vi "Image To Clipboard.vi"(8 "error in (no error)":errorcluster, 11 "24-bit pixmap":u32[][](array[numeric]) format="%x") -> (0 "error out":errorcluster)   [LabVIEW 2023, in "LV-Awesome.lvlib"]
uses:
  System.Drawing
  System.Windows.Forms
  LV-Awesome.lvlib
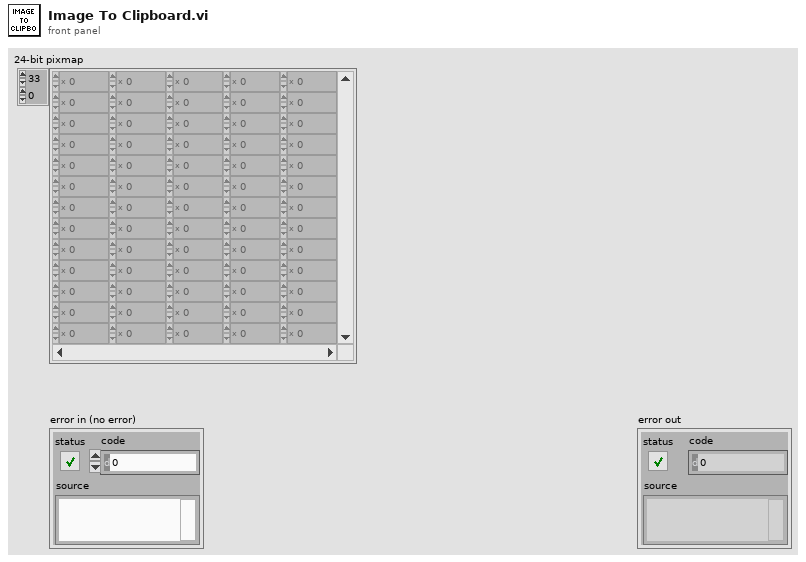
[diagram p1: front panel]
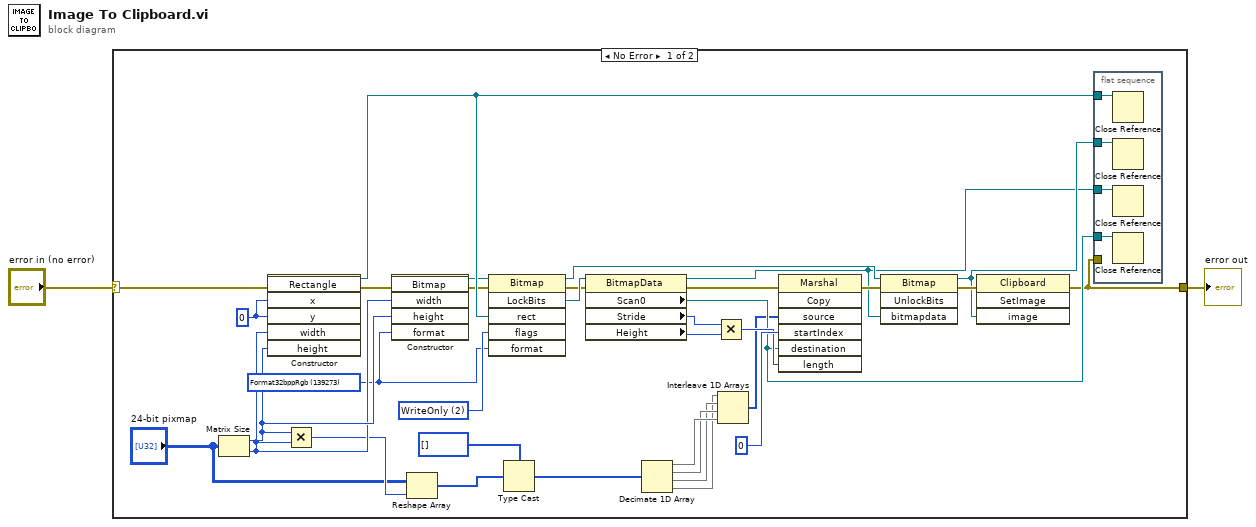
[diagram p0: block diagram]
diagram:
  n1 = case shown="No Error" "error in (no error)" {
    selector: "error in (no error)" -> [w11 w41]
    tunnel: [w10 w41] -> w1
    frame No Error {
      w35 = 2 items=["ReadOnly"=1, "WriteOnly"=2, "ReadWrite"=3, "UserInputBuffer"=4] ("flags")
      w36 = 0 ("x")
      w20 = 139273 items=["DontCare, Undefined"=0, "Max"=15, "Indexed"=65536, "Gdi"=131072, "Format16bppRgb555"=135173, "Format16bppRgb565"=135174, "Format24bppRgb"=137224, "Format32bppRgb"=139273, "Format1bppIndexed"=196865, "Format4bppIndexed"=197634, "Format8bppIndexed"=198659, "Alpha"=262144, "Format16bppArgb1555"=397319, "PAlpha"=524288, "Format32bppPArgb"=925707, "Extended"=1048576, "Format16bppGrayScale"=1052676, "Format48bppRgb"=1060876, "Format64bppPArgb"=1851406, "Canonical"=2097152, "Format32bppArgb"=2498570, "Format64bppArgb"=3424269] ("format")
      n2 = Matrix Size(0:"24-bit pixmap") -> (1:w32:i32, 2:w31:i32)
      n3 = constructor class="Rectangle"(error in=w11, "x"=w36, "y"=w36, "width"=w31, "height"=w32) -> (reference out=w13:refnum<k24>, error out=w25:errorcluster)  [unwired: 2 in, 5 out]
      n4 = Multiply(x=w32, y=w31) -> (x*y=w18:i32)
      n5 = constructor class="Bitmap"(error in=w25, "width"=w31, "height"=w32, "format"=w20) -> (reference out=w4:refnum<k24>, error out=w3:errorcluster)  [unwired: 2 in, 4 out]
      n6 = Reshape Array("24-bit pixmap", w18) -> (w19:u32[])
      n7 = invoke class="Bitmap" method="LockBits"(reference=w4, error in=w3, "rect"=w13, "flags"=w35, "format"=w20) -> (reference out=w28:refnum<k24>, error out=w26:errorcluster, "LockBits"=w34:refnum<k24>)  [unwired: 1 in, 3 out]
      n8 = Type Cast(type=u8[] [], x=w19) -> (*(type *) &x=w17:u8[])
      n9 = property class="BitmapData"(reference=w34, error in=w26) -> (reference out=w14:refnum<k24>, error out=w27:errorcluster, "Scan0"=w12:refnum<k24>, "Stride"=w22:i32, "Height"=w23:i32)
      n10 = Decimate 1D Array(w17) -> (w16:u8[], w7:u8[], w6:u8[], w5:u8[])
      n11 = Multiply(x=w22, y=w23) -> (x*y=w21:i32)
      n12 = Interleave 1D Arrays(w5, w6, w7, w16) -> (w8:u8[])
      n13 = invoke class="Marshal" method="Copy"(error in=w27, "source"=w8, "startIndex"=0, "destination"=w12, "length"=w21) -> (error out=w29:errorcluster)  [unwired: 2 in, 6 out]
      n14 = invoke class="Bitmap" method="UnlockBits"(reference=w28, error in=w29, "bitmapdata"=w14) -> (reference out=w15:refnum<k24>, error out=w24:errorcluster)  [unwired: 1 in, 2 out]
      n15 = invoke class="Clipboard" method="SetImage"(error in=w24, "image"=w15) -> (error out=w10:errorcluster)  [unwired: 2 in, 3 out]
      n16 = flat-sequence {
        tunnel: w10 -> [_]
        tunnel: w15 -> [w40]
        tunnel: w14 -> [w39]
        tunnel: w13 -> [w38]
        tunnel: w12 -> [w37]
        frame #0 {
          n17 = Close Reference(reference=w38) -> ()  [unwired: 1 in, 1 out]
          n18 = Close Reference(reference=w40) -> ()  [unwired: 1 in, 1 out]
          n19 = Close Reference(reference=w39) -> ()  [unwired: 1 in, 1 out]
          n20 = Close Reference(reference=w37) -> ()  [unwired: 1 in, 1 out]
        }
      }
    }
    frame Error {
    }
  }
  "error out" <- w1
